vi "Clocks.vi"() -> ()   [LabVIEW 2012]
panel:
  out "Numeric":dbl format="%02.0f"
  out "Numeric 2":dbl format="%0#2.0f"
  out "M 3":dbl(knob) scale=0.0..60.0
  out "H 3":dbl(knob) scale=0.0..60.0
  out "S 3":dbl(knob) scale=0.0..12.0
  out "M 2":dbl(knob) scale=0.0..60.0
  out "H 2":dbl(knob) scale=0.0..60.0
  out "S 2":dbl(knob) scale=0.0..12.0
  out "H":dbl(knob) scale=0.0..12.0
  out "M":dbl(knob) scale=0.0..60.0
  out "S":dbl(knob) scale=0.0..12.0
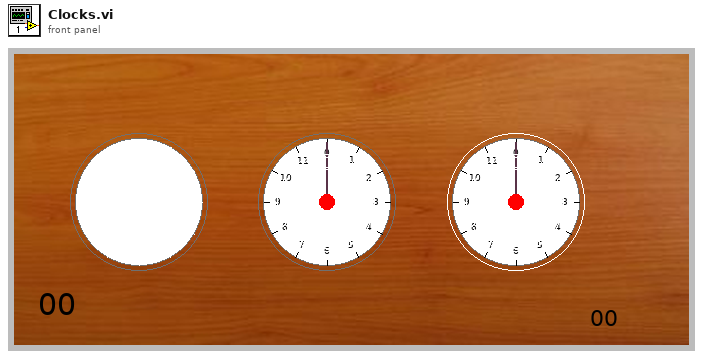
[diagram p1: front panel]
types:
  T1 = cluster{"second":i32, "minute":i32, "hour":i32, "day of month":i32, "month":i32, "year":i32, "day of week":i32, "day of year":i32, "is DST":i32}
  T2 = cluster{"second":dbl, "minute":dbl, "hour":dbl, "day of month":dbl, "month":dbl, "year":dbl, "day of week":dbl, "day of year":dbl, "is DST":dbl}
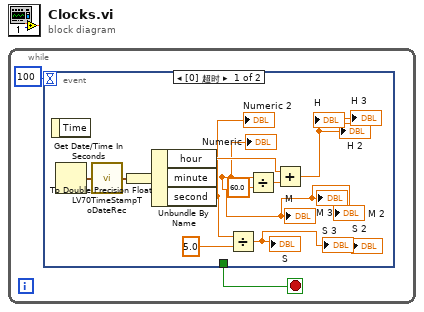
[diagram p0: block diagram]
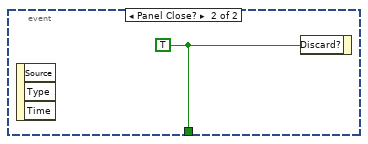
[diagram p2: hidden frame]
diagram:
  n1 = while {
    stop <- w1 stop-if-true
    n2 = event shown="[0] 超时" {
      selector: _ -> [_ _]
      dyn-events: _ -> [_ _]
      timeout: 100 -> [_ _]
      tunnel: [_ w14] -> w1
      event Timeout {
        n3 = event-data() -> ()  [unwired: 1 in, 1 out]
        n4 = Get Date/Time In Seconds() -> (seconds since 1Jan1904=w13:timestamp)
        n5 = call <vilib>:"LV70TimeStampToDateRec.vi"("time stamp"=w13) -> ("date time rec"=w12:T1)
        n6 = To Double Precision Float(number=w12) -> (double precision float=w7:T2)
        n7 = Unbundle By Name(w7) -> ("hour"=w8:dbl, "minute"=w3:dbl, "second"=w4:dbl)
        "M" <- w3
        "M 3" <- w3
        "M 2" <- w3
        "Numeric 2" <- w4
        "Numeric" <- w3
        n8 = Divide(x=w4, y=5.0) -> (x/y=→"S" →"S 3" →"S 2":dbl)
        n9 = Divide(x=w3, y=60.0) -> (x/y=w9:dbl)
        n10 = Add(x=w8, y=w9) -> (x+y=→"H" →"H 3" →"H 2":dbl)
      }
      event Panel Close? {
        w14 = TRUE
        n11 = event-data() -> ()  [unwired: 1 in, 3 out]
        n12 = event-data("Discard?"=w14) -> ()  [unwired: 1 in, 1 out]
      }
    }
  }
